vi "Write Width.vi"(8 "error in (no error)":errorcluster, 10 "Width":u32, 11 "ActiveXContainer in":refnum<class "ActiveXContainer.lvclass">) -> (0 "error out":errorcluster, 3 "ActiveXContainer out":refnum<class "ActiveXContainer.lvclass">)   [LabVIEW 2020, in "WebView2 QControl.lvlib" / "ActiveXContainer.lvclass"]
uses:
  ActiveXContainer.lvclass
  ActiveXContainer.lvclass/ActiveXContainer.ctl
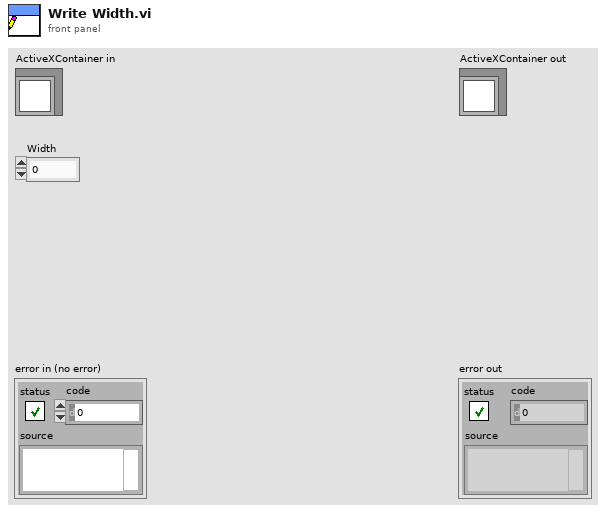
[diagram p1: front panel]
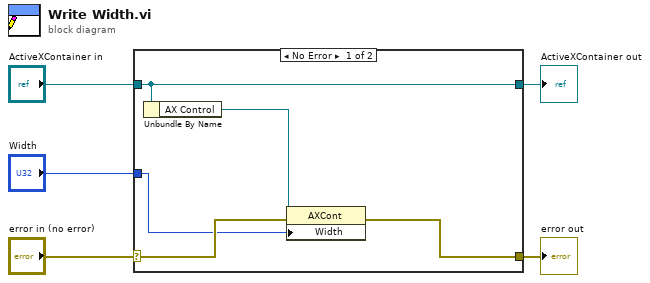
[diagram p0: block diagram]
diagram:
  n1 = case shown="No Error" "error in (no error)" {
    selector: "error in (no error)" -> [w10 w11]
    tunnel: [w8 w11] -> w4
    tunnel: [w9 w12] -> w2
    tunnel: "ActiveXContainer in" -> [w9 w12]
    tunnel: "Width" -> [w6 _]
    frame No Error {
      n2 = Unbundle By Name(w9) -> ("AX Control"=w7:refnum<vi>)
      n3 = property class="AXCont"(reference=w7, error in=w10, "Width"=w6) -> (error out=w8:errorcluster)  [unwired: 1 out]
    }
    frame Error {
    }
  }
  "error out" <- w4
  "ActiveXContainer out" <- w2
